vi "Parse Files.vi"(8 "error in (no error)":errorcluster, 11 "LVProject in":refnum<class "LVProject.lvclass">) -> (0 "error out":errorcluster, 3 "LVProject out":refnum<class "LVProject.lvclass">)   [LabVIEW 2020, in "GPack.lvlib" / "LVProject.lvclass"]
uses:
  LVProject.lvclass
  LVProject.lvclass/LVProject.ctl
  <vilib>/xml/Close Reference(Node).vi
  <vilib>/xml/NI_XML.lvlib
panel:
  out "Array":T1(array[cluster])
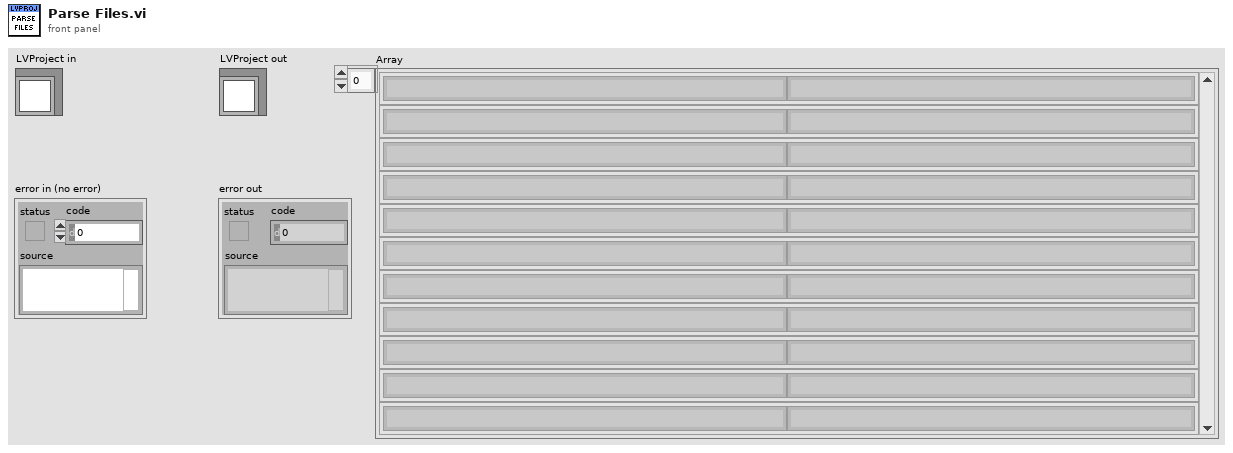
[diagram p1: front panel]
types:
  T1 = cluster{"node text":string, "OS Path String":string}[]
  T2 = cluster{"node text":string, "OS Path String":string}
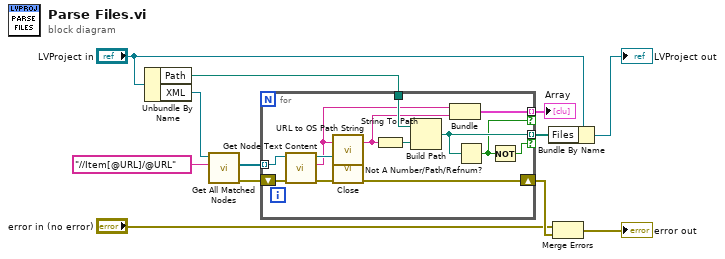
[diagram p0: block diagram]
diagram:
  n1 = Unbundle By Name("LVProject in") -> ("Path"=w5:path, "XML"=w1:refnum<k20>)
  n2 = call <vilib>:"Get All Matched Nodes.vi"("XPath expression"="//Item[@URL]/@URL", "node in"=w1) -> ("error out"=w8:errorcluster, "node result array"=w2:refnum<k20>[])  [unwired: 7 in, 1 out]
  n3 = for {
    tunnel: w2 -> [w22] mode=indexing
    shift-right: [w19] -> w12
    shift-left: w8 -> [w23]
    tunnel: w5 -> [w24]
    tunnel: [w18] -> w4 mode=indexing if=w14
    tunnel: [w16] -> w3 mode=indexing if=w15
    n4 = call <vilib>:"Get Node Text Content.vi"("error in (no error)"=w23, "node in"=w22) -> ("error out"=w20:errorcluster, "node text"=w13:string, "node out"=w21:refnum<k20>)  [unwired: 7 in]
    n5 = call "URL to OS Path String.vi"("URL Path String"=w13) -> ("OS Path String"=w17:string)  [unwired: 2 in]
    n6 = call-poly <vilib>:"Close.vi"("error in (no error)"=w20, "node"=w21) -> ("error out"=w19:errorcluster)  [unwired: 7 in]
    n7 = String To Path(string=w17) -> (path=w25:path)
    n8 = Build Path(base path=w24, name or relative path=w25) -> (appended path=w18:path)
    n9 = Bundle("node text"=w13, "OS Path String"=w17) -> (w16:T2)  [unwired: 1 in]
    n10 = Not A Number/Path/Refnum?(number/path/refnum=w18) -> (NaN/Path/Refnum?=w15:bool)
    n11 = Not(x=w15) -> (.not. x?=w14:bool)
  }
  "Array" <- w3
  n12 = Bundle By Name(cluster="LVProject in", "Files"=w4) -> (→"LVProject out":refnum<class "LVProject.lvclass">)
  n13 = Merge Errors("error in (no error)", w12) -> (→"error out":errorcluster)
